vi "Analysis GUI.vi"(9 "Remote Path":path=path "d:/testdata/temp", 10 "Results Path":path=path "c:/testdata/TestResults", 11 "Temp Path":path=path "c:/testdata/temp") -> ()   [LabVIEW 2014, in "NIAnalysis.lvlib"]
uses:
  NIAnalysis.lvlib
  Types/AnalysisGUI.Refs.ctl
panel:
  out "Cycle":i32
  in  "error in (no error)":errorcluster
  out "Cycle Result":string
  in  "Stop":bool
  out "Results Directory":path=path "d:/testdata/TestResults"
  out "Data File":path
  in  "Tree":string(tree)
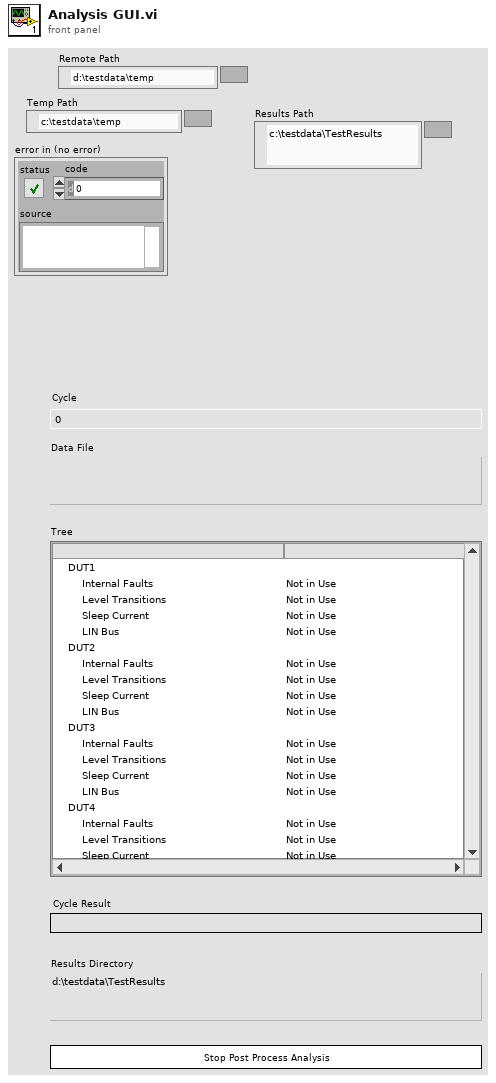
[diagram p1: front panel]
types:
  T1 = typedef "NIAnalysis.lvlib/AnalysisGUI.Refs.ctl" = cluster{"Data File":refnum<vi>, "Cycle":refnum<vi>, "Cycle Result":refnum<vi>, "Tree":refnum<vi>}
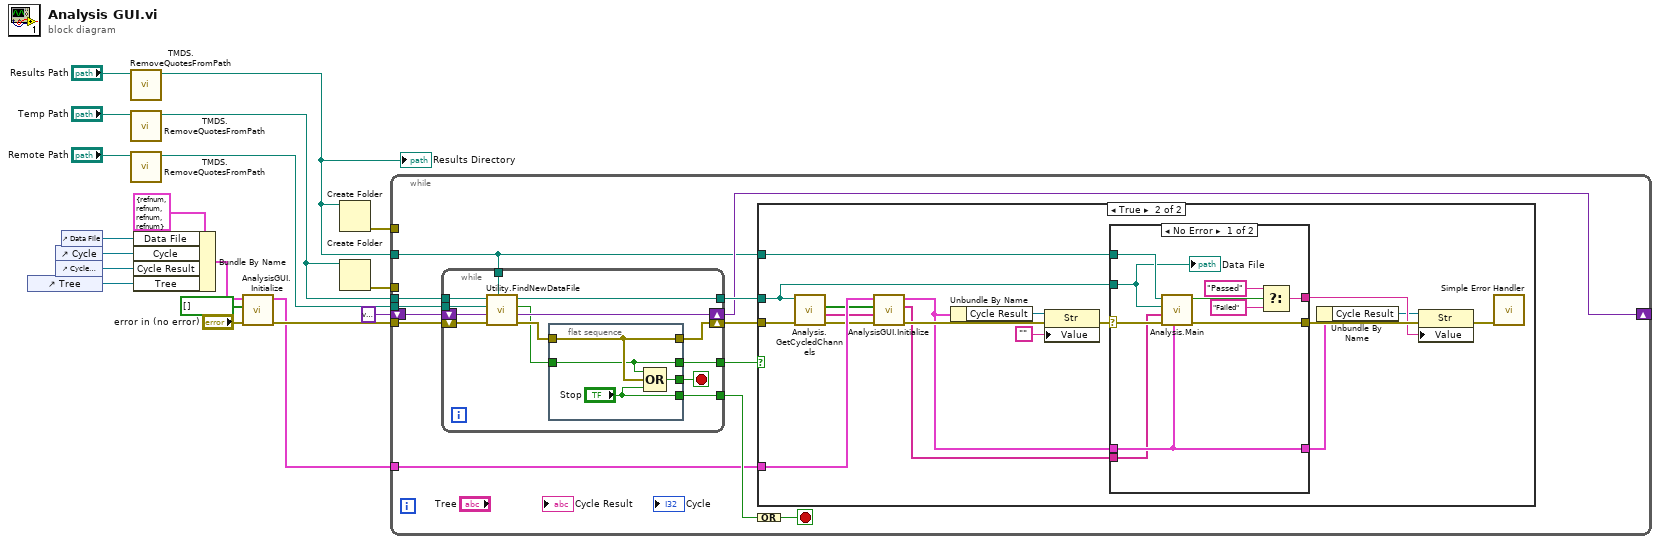
[diagram p0: block diagram]
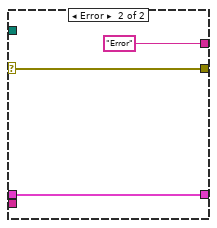
[diagram p3: hidden frame]
diagram:
  n1 = control-ref of="Tree"() -> (w14:refnum<vi>)
  n2 = control-ref of="Cycle"() -> (w12:refnum<vi>)
  n3 = control-ref of="Cycle Result"() -> (w17:refnum<vi>)
  n4 = control-ref of="Data File"() -> (w18:refnum<vi>)
  n5 = call "TMDS.RemoveQuotesFromPath.vi"("Data"="Results Path") -> ("Path"=w4:path)  [unwired: 9 in, 1 out]
  "Results Directory" <- w4
  n6 = call "TMDS.RemoveQuotesFromPath.vi"("Data"="Temp Path") -> ("Path"=w3:path)  [unwired: 9 in, 1 out]
  n7 = call "TMDS.RemoveQuotesFromPath.vi"("Data"="Remote Path") -> ("Path"=w7:path)  [unwired: 9 in, 1 out]
  n8 = Bundle By Name(cluster=T1 {"Data File"=refnum, "Cycle"=refnum, "Cycle Result"=refnum, "Tree"=refnum} ("output cluster"), "Data File"=w18, "Cycle"=w12, "Cycle Result"=w17, "Tree"=w14) -> (w15:T1)
  n9 = call "AnalysisGUI.Initialize.vi"("error in (no error)"="error in (no error)", "Use?"=bool[] [], "Refs"=w15) -> ("error out"=w19:errorcluster, "Refs"=w11:T1)  [unwired: 6 in, 1 out]
  n10 = Create Folder(path (use dialog)=w4) -> (error out=w2:errorcluster)  [unwired: 2 in, 2 out]
  n11 = Create Folder(path (use dialog)=w3) -> (error out=w1:errorcluster)  [unwired: 2 in, 2 out]
  n12 = while {
    tunnel: w19 -> [w28]
    tunnel: w3 -> [w31]
    tunnel: w4 -> [w21]
    tunnel: w11 -> [w27]
    shift-right: [w24] -> _
    shift-left: variant -> [w25]
    tunnel: w7 -> [w20]
    tunnel: w2 -> [_]
    tunnel: w1 -> [_]
    stop <- w29 stop-if-true
    n13 = while {
      tunnel: w31 -> [w75]
      shift-right: [w72] -> w23
      shift-left: w28 -> [w74]
      tunnel: [w65] -> w26
      tunnel: [w71] -> w22
      tunnel: [w69] -> w30
      shift-right: [w67] -> w24
      shift-left: w25 -> [w68]
      tunnel: w21 -> [w64]
      tunnel: w20 -> [w63]
      stop <- w70 stop-if-true
      n14 = call "Utility.FindNewDataFile.vi"("Results Path"=w64, "error in (no error)"=w74, "LookupTable"=w68, "Remote Path"=w63, "Path"=w75) -> ("error out"=w73:errorcluster, "LookupTable out"=w67:variant, "Found"=w66:bool, "path out"=w65:path)  [unwired: 3 in]
      n15 = flat-sequence {
        tunnel: w66 -> [w76]
        tunnel: [w79] -> w70
        tunnel: w73 -> [w78]
        tunnel: [w78] -> w72
        tunnel: [w76] -> w71
        tunnel: ["Stop"] -> w69
        frame #0 {
          n16 = Compound Arithmetic op=OR(w76, w78, "Stop") -> (w79:bool)
        }
      }
    }
    n17 = case shown="True" w22 {
      tunnel: w21 -> [_ w49]
      tunnel: w27 -> [_ w40]
      tunnel: w26 -> [_ w39]
      tunnel: w23 -> [_ w34]
      frame False {
      }
      frame True {
        n18 = call "Analysis.GetCycledChannels.vi"("error in (no error)"=w34, "Data"=w39) -> ("error out"=w38:errorcluster, "DUTs"=w33:string[], "Cycled"=w37:bool[])  [unwired: 7 in]
        n19 = call "AnalysisGUI.Initialize.vi"("error in (no error)"=w38, "DUTs"=w33, "Use?"=w37, "Refs"=w40) -> ("error out"=w42:errorcluster, "Tree Strings"=w32:string[], "Refs"=w41:T1)  [unwired: 5 in]
        n20 = Unbundle By Name(w41) -> ("Cycle Result"=w47:refnum<vi>)
        n21 = property class="Str"(reference=w47, error in=w42, "Value"="" ("Cycle Result")) -> (error out=w36:errorcluster)  [unwired: 1 out]
        n22 = case shown="No Error" w36 {
          selector: w36 -> [w58 w62]
          tunnel: w39 -> [w51 _]
          tunnel: w49 -> [w57 _]
          tunnel: [w59 w62] -> w48
          tunnel: w41 -> [w52 w60]
          tunnel: [w53 "Error"] -> w45
          tunnel: [w52 w60] -> w44
          tunnel: w32 -> [w50 _]
          frame No Error {
            n23 = call "Analysis.Main.vi"("Refs"=w52, "error in (no error)"=w58, "Headers"=w50, "Data Path"=w51, "Result Directory"=w57) -> ("error out"=w59:errorcluster, "Overall Result"=w54:bool)  [unwired: 5 in]
            n24 = Select(t="Passed", s=w54, f="Failed") -> (s? t:f=w53:string)
            "Data File" <- w51
          }
          frame Error {
          }
        }
        n25 = Unbundle By Name(w44) -> ("Cycle Result"=w43:refnum<vi>)
        n26 = property class="Str"(reference=w43, error in=w48, "Value"=w45) -> (error out=w35:errorcluster)  [unwired: 1 out]
        n27 = call <vilib>:"Simple Error Handler.vi"("error in (no error)"=w35) -> ()  [unwired: 4 in, 5 out]
      }
    }
    n28 = Compound Arithmetic op=OR(w30) -> (w29:bool)
  }
